vi "TimeInterpPose_AddSample.vi"(9 "Pose":T1={"TRANSLATION"={"X"=0.0, "Y"=0.0}, "ROTATION"={"VALUE"=0.0, "COS"=1.0, "SIN"=0.0}} {"ROTATION"."SIN" format="%13.4f"; "ROTATION"."COS" format="%13.4f"; "ROTATION"."VALUE" format="%13.4f"; "TRANSLATION"."Y" format="%14.3f"; "TRANSLATION"."X" format="%14.3f"}, 10 "TimeStamp":dbl, 11 "in TimeInterpPose":T4 {"Pose"."ROTATION"."SIN" format="%13.4f"; "Pose"."ROTATION"."COS" format="%13.4f"; "Pose"."ROTATION"."VALUE" format="%13.4f"; "Pose"."TRANSLATION"."Y" format="%14.3f"; "Pose"."TRANSLATION"."X" format="%14.3f"}) -> (3 "out TimeInterpPose":T4 {"Pose"."ROTATION"."SIN" format="%13.4f"; "Pose"."ROTATION"."COS" format="%13.4f"; "Pose"."ROTATION"."VALUE" format="%13.4f"; "Pose"."TRANSLATION"."Y" format="%14.3f"; "Pose"."TRANSLATION"."X" format="%14.3f"})   [LabVIEW 2019, in "Trajectory_Library.lvlib"]
doc: "Insert new X, Y pair into an existing Function Generator data cluster.\n\nInputs:\n - \n\nOutputs:\n - Function Generator -- Created data structure"
uses:
  Trajectory_Library.lvlib
  TIME_INTERPOLATABLE_POSE.ctl
  POSE2D.ctl
  TRANSLATION2D.ctl
  ROTATION2D.ctl
  <vilib>/gmath/NI_Gmath.lvlib
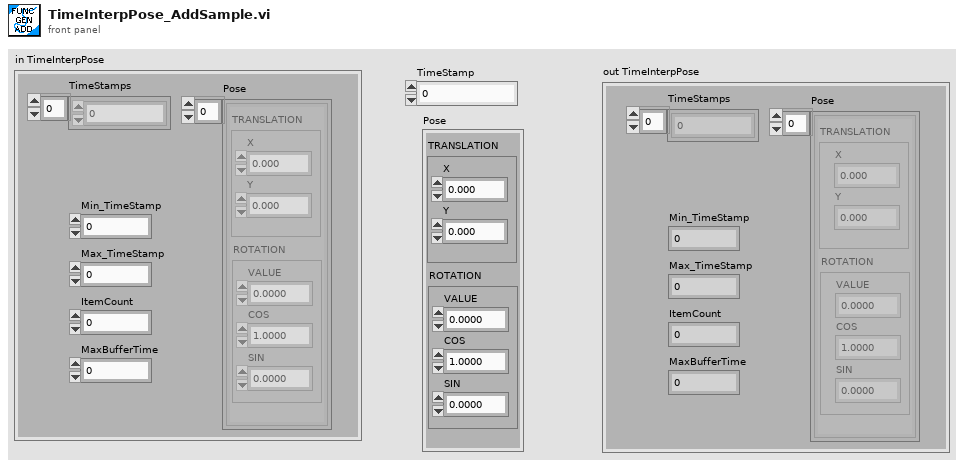
[diagram p1: front panel]
types:
  T1 = typedef "Trajectory_Library.lvlib/POSE2D.ctl" = cluster{"TRANSLATION":T2, "ROTATION":T3}
  T2 = typedef "Trajectory_Library.lvlib/TRANSLATION2D.ctl" = cluster{"X":dbl, "Y":dbl}
  T3 = typedef "Trajectory_Library.lvlib/ROTATION2D.ctl" = cluster{"VALUE":dbl, "COS":dbl, "SIN":dbl}
  T4 = typedef "Trajectory_Library.lvlib/TIME_INTERPOLATABLE_POSE.ctl" = cluster{"TimeStamps":dbl[], "Pose":T1[], "Min_TimeStamp":dbl, "Max_TimeStamp":dbl, "ItemCount":i32, "MaxBufferTime":dbl}
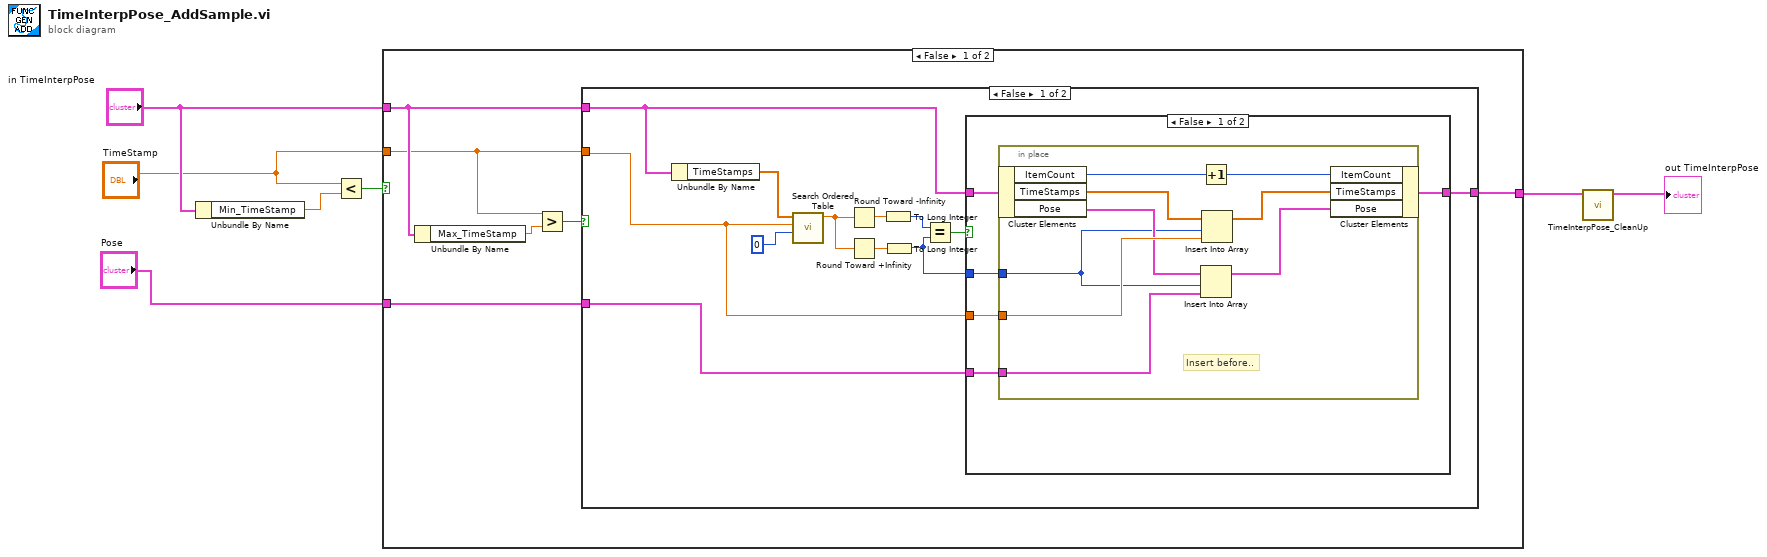
[diagram p0: block diagram]
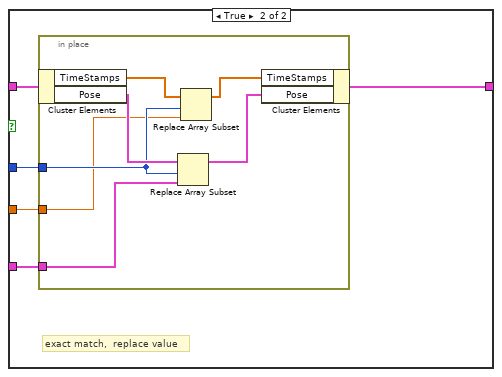
[diagram p2: hidden frame]
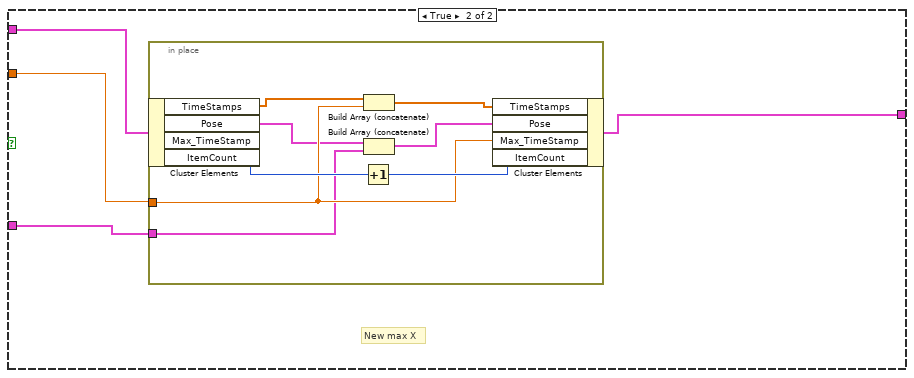
[diagram p3: hidden frame]
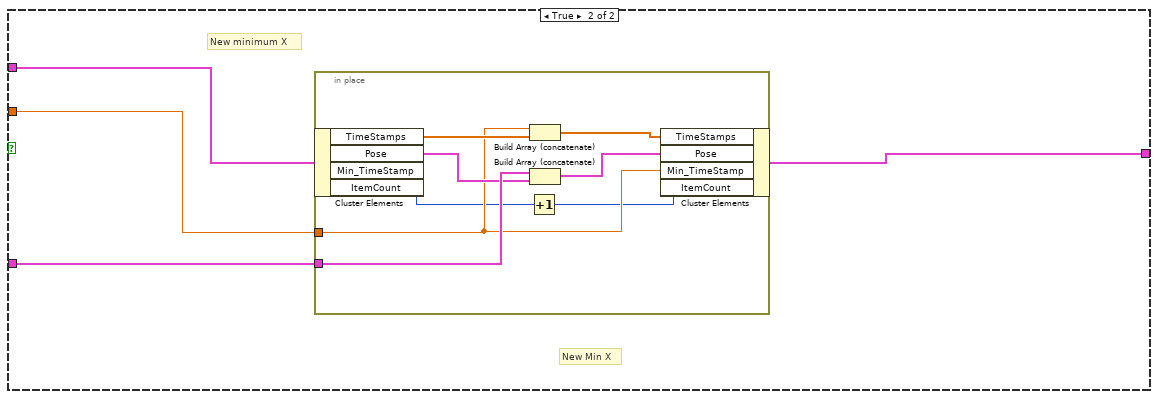
[diagram p4: hidden frame]
diagram:
  n1 = Unbundle By Name("in TimeInterpPose") -> ("Min_TimeStamp"=w7:dbl)
  n2 = Less?(x="TimeStamp", y=w7) -> (x < y?=w6:bool)
  n3 = case shown="False" w6 {
    tunnel: "in TimeInterpPose" -> [w11 w67]
    tunnel: "TimeStamp" -> [w9 w66]
    tunnel: "Pose" -> [w8 w65]
    tunnel: [w10 w64] -> w2
    frame False {
      n4 = Unbundle By Name(w11) -> ("Max_TimeStamp"=w13:dbl)
      n5 = Greater?(x=w9, y=w13) -> (0:w12:bool)
      n6 = case shown="False" w12 {
        tunnel: w11 -> [w18 w55]
        tunnel: [w14 w54] -> w10
        tunnel: w9 -> [w16 w53]
        tunnel: w8 -> [w15 w52]
        frame False {
          n7 = Unbundle By Name(w18) -> ("TimeStamps"=w24:dbl[])
          n8 = call <vilib>:"Search Ordered Table.vi"("starting index"=0, "x value"=w16, "ordered x array"=w24) -> ("fractional index"=w23:dbl)  [unwired: 8 in]
          n9 = Round Toward -Infinity(1:w23) -> (0:w21:dbl)
          n10 = Round Toward +Infinity(x=w23) -> (ceil(x): smallest int >= x=w22:dbl)
          n11 = To Long Integer(number=w21) -> (32bit integer=w20:i32)
          n12 = To Long Integer(number=w22) -> (32bit integer=w17:i32)
          n13 = Equal?(x=w20, y=w17) -> (x = y?=w19:bool)
          n14 = case shown="False" w19 {
            tunnel: w18 -> [w27 w44]
            tunnel: w17 -> [w30 w43]
            tunnel: w16 -> [w29 w42]
            tunnel: w15 -> [w28 w41]
            tunnel: [w26 w40] -> w14
            frame False {
              n15 = in-place {
                in-place-border: w30 -> [w34]
                in-place-border: w29 -> [w36]
                in-place-border: w28 -> [w33]
                # "Insert before.."
                n16 = in-place-cluster #1(w27) -> ("ItemCount"=w39:i32, "TimeStamps"=w37:dbl[], "Pose"=w35:T1[])
                n17 = Increment(x=w39) -> (x+1=w38:i32)
                n18 = Insert Into Array(array=w35, index=w34, new element=w33) -> (w31:T1[])
                n19 = Insert Into Array(array=w37, index=w34, new element=w36) -> (w32:dbl[])
                n20 = in-place-cluster #1("ItemCount"=w38, "TimeStamps"=w32, "Pose"=w31) -> (w26:T4)
              }
            }
            frame True {
              # "exact match,  replace value"
              n21 = in-place {
                in-place-border: w43 -> [w49]
                in-place-border: w42 -> [w48]
                in-place-border: w41 -> [w47]
                n22 = in-place-cluster #2(w44) -> ("TimeStamps"=w51:dbl[], "Pose"=w50:T1[])
                n23 = Replace Array Subset(array=w50, new element=w47, index=w49) -> (w45:T1[])
                n24 = Replace Array Subset(array=w51, new element=w48, index=w49) -> (w46:dbl[])
                n25 = in-place-cluster #2("TimeStamps"=w46, "Pose"=w45) -> (w40:T4)
              }
            }
          }
        }
        frame True {
          # "New max X"
          n26 = in-place {
            in-place-border: w53 -> [w59]
            in-place-border: w52 -> [w56]
            n27 = in-place-cluster #3(w55) -> ("TimeStamps"=w58:dbl[], "Pose"=w57:T1[], "ItemCount"=w61:i32)  [unwired: 1 out]
            n28 = Increment(x=w61) -> (x+1=w60:i32)
            n29 = Build Array (concatenate)(w58, w59) -> (w63:dbl[])
            n30 = Build Array (concatenate)(w57, w56) -> (w62:T1[])
            n31 = in-place-cluster #3("TimeStamps"=w63, "Pose"=w62, "Max_TimeStamp"=w59, "ItemCount"=w60) -> (w54:T4)
          }
        }
      }
    }
    frame True {
      # "New Min X"
      # "New minimum X"
      n32 = in-place {
        in-place-border: w66 -> [w70]
        in-place-border: w65 -> [w75]
        n33 = in-place-cluster #4(w67) -> ("TimeStamps"=w74:dbl[], "Pose"=w71:T1[], "ItemCount"=w69:i32)  [unwired: 1 out]
        n34 = Increment(x=w69) -> (x+1=w68:i32)
        n35 = Build Array (concatenate)(w70, w74) -> (w73:dbl[])
        n36 = Build Array (concatenate)(w75, w71) -> (w72:T1[])
        n37 = in-place-cluster #4("TimeStamps"=w73, "Pose"=w72, "Min_TimeStamp"=w70, "ItemCount"=w68) -> (w64:T4)
      }
    }
  }
  n38 = call "TimeInterpPose_CleanUp.vi"("in TimeInterpPose"=w2) -> ("out TimeInterpPose"=→"out TimeInterpPose":T4)  [unwired: 10 in]
